vi "Get Reference Target Name.vi"(11 "Project Sync Tools in":refnum<class "Project Sync Tools.lvclass">) -> (2 "Reference Target Name":string, 3 "Project Sync Tools out":refnum<class "Project Sync Tools.lvclass">)   [LabVIEW 2019, in "Project Sync Tools.lvclass"]
uses:
  Project Sync Tools.lvclass
  Project Sync Tools.lvclass/Project Sync Tools.ctl
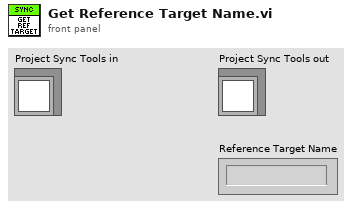
[diagram p1: front panel]
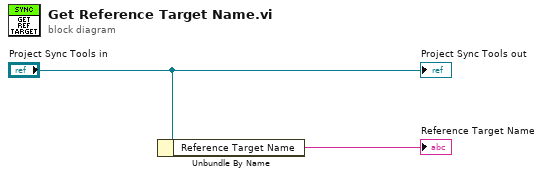
[diagram p0: block diagram]
diagram:
  n1 = Unbundle By Name("Project Sync Tools in") -> ("Reference Target Name"=→"Reference Target Name":string)
  "Project Sync Tools out" <- "Project Sync Tools in"
